vi "getUserEvent.vi"(8 "error in (no error)":errorcluster, 11 "ForecastDisplay in":refnum<class "ForecastDisplay.lvclass">) -> (0 "error out":errorcluster, 2 "UserEvent":refnum<user-event>, 3 "ForecastDisplay out":refnum<class "ForecastDisplay.lvclass">)   [LabVIEW 2018, in "ForecastDisplay.lvclass"]
uses:
  ForecastDisplay.lvclass
  Observer/Observer.lvclass
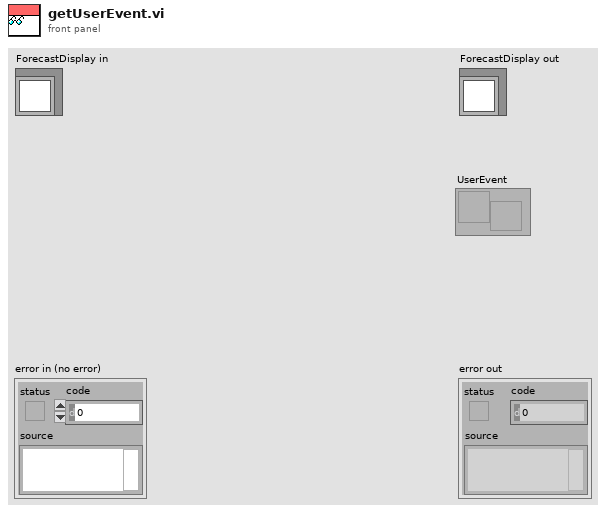
[diagram p1: front panel]
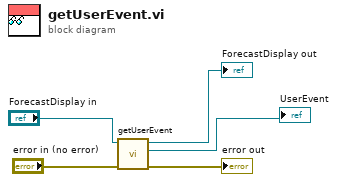
[diagram p0: block diagram]
diagram:
  n1 = call-parent "getUserEvent.vi"("error in (no error)"="error in (no error)", "Observer in"="ForecastDisplay in") -> ("error out"=→"error out":errorcluster, "UserEvent"=→"UserEvent":refnum<user-event>, "Observer out"=→"ForecastDisplay out":refnum<class "ForecastDisplay.lvclass">)  [unwired: 7 in]
